vi "TDK多功能.vi"(0 "TDK地址":refnum<visa-resource-name>="COM15", 1 "工况1循环次数":i32, 2 "电源台数":dbl=3.0, 3 "工况1":string, 5 "工况切换地址":refnum<visa-resource-name>, 7 "工况2循环次数":i32, 9 "字符串":string, 10 "大循环次数":i32, 11 "错误输入（无错误）":errorcluster, 12 "工况地址":path, 13 "Bool引用句柄":refnum<vi>, 14 "工况2":string) -> (4 "运行总时间":dbl, 15 "错误输出":errorcluster)   [LabVIEW 2021]
uses:
  <vilib>/Utility/file.llb/Read Delimited Spreadsheet (DBL).vi
panel:
  out "?":string
  out "已成大循环数":i32
  in  "工况2":u16(ring) items=["新建 文本文档 (2)", "新建 文本文档 (3)", "新建 文本文档 (4)", "新建 文本文档"]
  in  "工况1":u16(ring) items=["新建 文本文档 (2)", "新建 文本文档 (3)", "新建 文本文档 (4)", "新建 文本文档"]
  out "?":u8(slide) scale=0.0..100.0
  out "电流":dbl(knob) scale=0.0..2000.0
  out "?":dbl[](graph)
  out "完成工况2循环":i32
  out "完成工况1循环":i32
  in  "延迟时间":dbl=1.0 caption="延迟时间(s)"
  in  "输入电流(A)":dbl
  in  "电流方向控制":cluster{"正向":bool, "反向":bool}
  out "?":bool
  out "?":bool
  in  "工况1":string[][](table)
  in  "工况2":string[][](table)
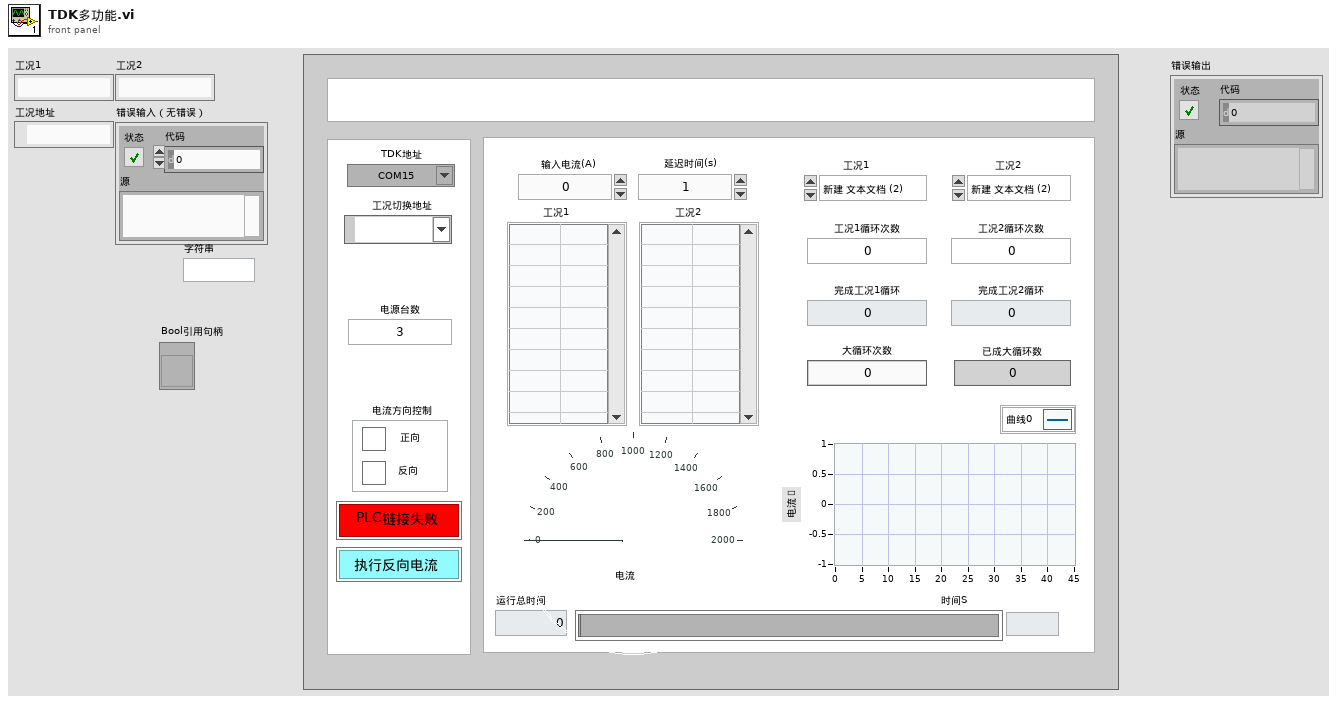
[diagram p1: front panel]
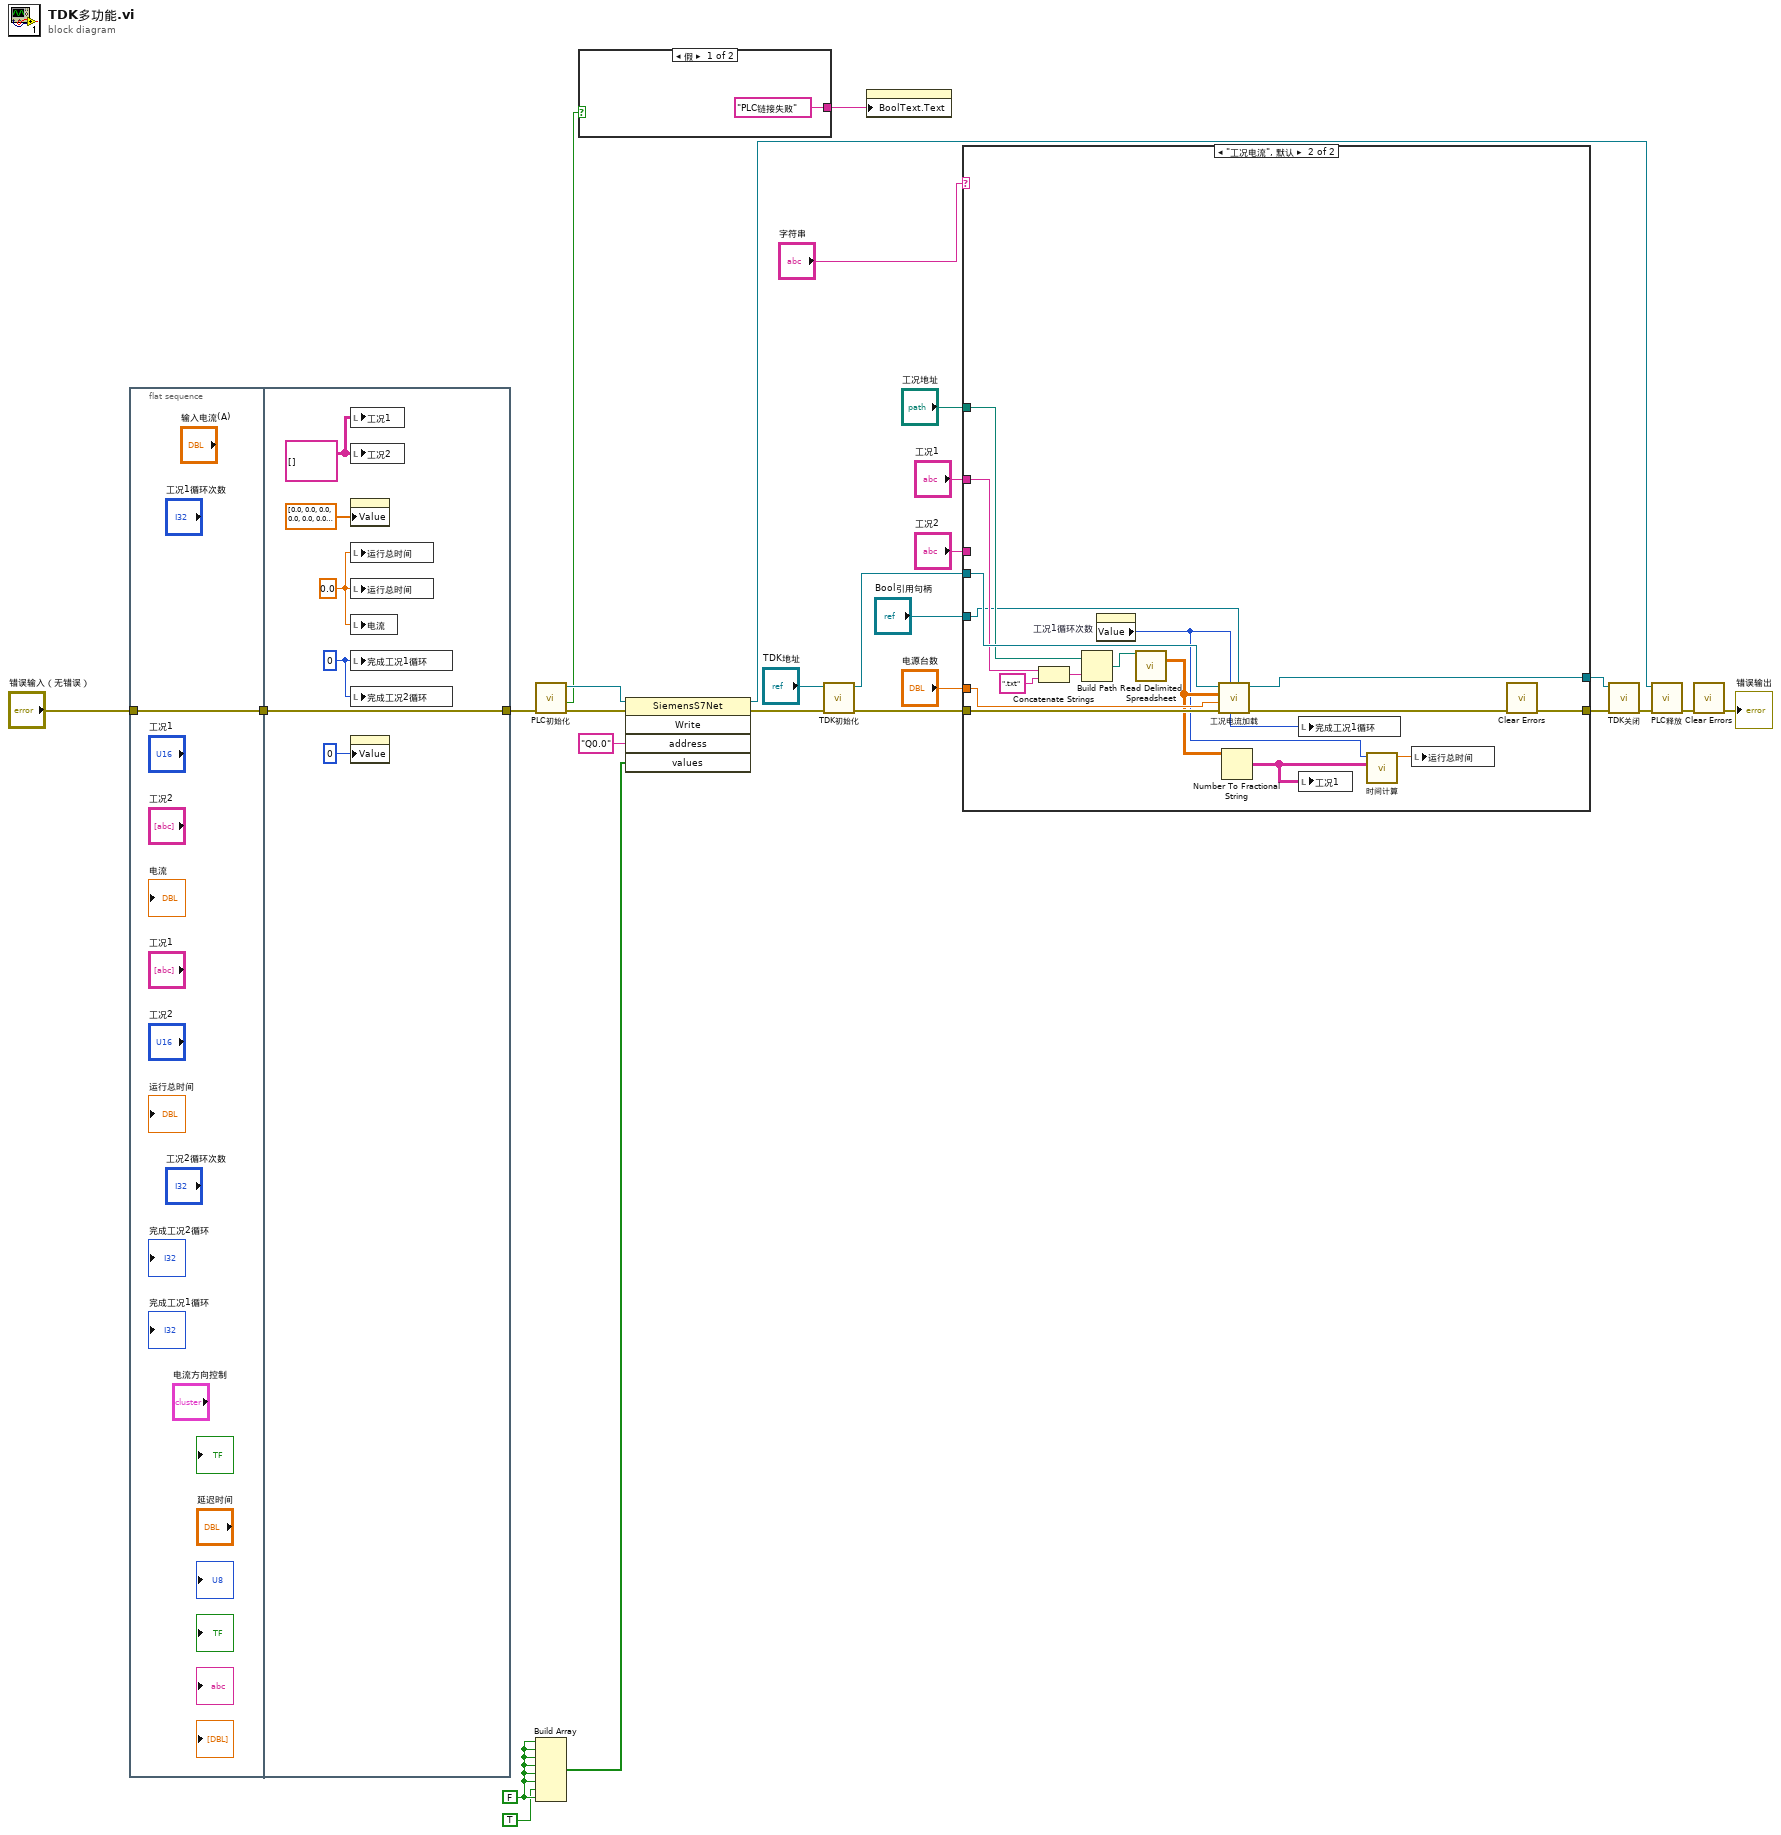
[diagram p0: block diagram]
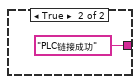
[diagram p2: hidden frame]
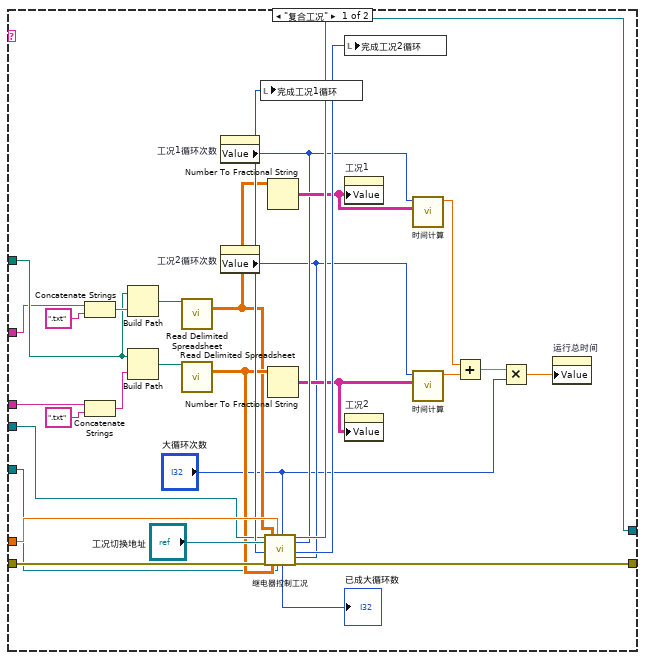
[diagram p3: hidden frame]
diagram:
  w11 = FALSE ("停止")
  n1 = flat-sequence {
    tunnel: "错误输入（无错误）" -> [w28]
    tunnel: [w28] -> w14
    tunnel: [w31] -> w8
    tunnel: w14 -> [w31]
    frame #0 {
    }
    frame #1 {
      w33 = 0
      w34 = string[][] [] ("工况1")
      w30 = 0.0
      n2 = local write "工况1"(w34) -> ()
      n3 = local write "工况2"(w34) -> ()
      n4 = property class="WFGraph (严格)"("Value"=dbl[] [0.0, 0.0, 0.0, 0.0, 0.0, 0.0, 0.0, 0.0, 0.0, 0.0, 0.0, 0.0, 0.0, 0.0, 0.0, 0.0, 0.0, 0.0, 0.0, 0.0, 0.0, 0.0, 0.0, 0.0, 0.0, 0.0, 0.0, 0.0, 0.0, 0.0, 0.0, 0.0, 0.0, 0.0, 0.0, 0.0, 0.0, 0.0, 0.0, 0.0, 0.0, 0.0, 0.0, 0.0, 0.0, 0.0]) -> ()  [unwired: 2 in, 2 out]
      n5 = local write "运行总时间"(w30) -> ()
      n6 = local write "运行总时间"(w30) -> ()
      n7 = local write "电流"(w30) -> ()
      n8 = local write "完成工况1循环"(w33) -> ()
      n9 = local write "完成工况2循环"(w33) -> ()
      n10 = property class="Slide (严格)"("Value"=u8 0) -> ()  [unwired: 2 in, 2 out]
    }
  }
  n11 = call "PLC初始化.vi"("错误输入（无错误）"=w8) -> ("错误输出"=w25:errorcluster, "IsSuccess"=w17:bool, "引用输出"=w26:refnum<k24>)  [unwired: 8 in]
  n12 = Build Array(w11, w11, w11, w11, w11, w11, TRUE ("元素"), w11) -> (w23:bool[])
  n13 = case shown="假" w17 {
    tunnel: ["PLC链接失败" "PLC链接成功"] -> w16
    frame False {
    }
    frame True {
    }
  }
  n14 = invoke class="SiemensS7Net" method="Write"(reference=w26, error in=w25, "address"="Q0.0", "values"=w23) -> (reference out=w20:refnum<k24>, error out=w24:errorcluster)  [unwired: 1 in, 3 out]
  n15 = call "TDK初始化.vi"("error in (no error)"=w24, "TDK地址"="TDK地址") -> ("error out"=w13:errorcluster, "VISA resource name out"=w15:refnum<visa-resource-name>)  [unwired: 8 in]
  n16 = property class="Bool (严格)"("BoolText.Text"=w16) -> ()  [unwired: 2 in, 2 out]
  n17 = case shown="\"工况电流\", 默认" "字符串" {
    tunnel: w15 -> [w58 w83]
    tunnel: [w62 w80] -> w18
    tunnel: w13 -> [w64 w81]
    tunnel: [w63 w74] -> w19
    tunnel: "电源台数" -> [w61 w82]
    tunnel: "工况地址" -> [w53 w77]
    tunnel: "工况1" -> [w39 w68]
    tunnel: "工况2" -> [w38 _]
    tunnel: "Bool引用句柄" -> [w37 w67]
    frame "复合工况" {
      n18 = Concatenate Strings(w39, ".txt" ("字符串")) -> (w54:string)
      n19 = Concatenate Strings(w38, ".txt" ("字符串")) -> (w57:string)
      n20 = Build Path(base path=w53, name or relative path=w54) -> (appended path=w50:path)
      n21 = Build Path(base path=w53, name or relative path=w57) -> (appended path=w52:path)
      n22 = call-poly <vilib>:"Read Delimited Spreadsheet.vi"("file path (dialog if empty)"=w50) -> ("all rows"=w49:dbl[][])  [unwired: 9 in, 5 out]
      n23 = call-poly <vilib>:"Read Delimited Spreadsheet.vi"("file path (dialog if empty)"=w52) -> ("all rows"=w51:dbl[][])  [unwired: 9 in, 5 out]
      n24 = property on="工况1循环次数" class="DigNum (严格)"() -> ("Value"=w47:i32)  [unwired: 2 in, 2 out]
      n25 = property on="工况2循环次数" class="DigNum (严格)"() -> ("Value"=w45:i32)  [unwired: 2 in, 2 out]
      n26 = call "继电器控制工况.vi"("tdk"=w58, "6332b"="工况切换地址", "error out"=w64, "工况1"=w49, "工况2"=w51, "电源台数"=w61, "Bool引用句柄"=w37, "大循环次数"="大循环次数", "工况1循环次数"=w47, "工况2循环次数"=w45) -> ("完成工况1循环"=w60:i32, "已成大循环数"=→"已成大循环数":i32, "VISA resource name out"=w62:refnum<visa-resource-name>, "完成工况2循环"=w59:i32, "错误输出"=w63:errorcluster)  [unwired: 5 in]
      n27 = local write "完成工况1循环"(w60) -> ()
      n28 = Number To Fractional String(number=w49) -> (F-format string=w48:string[][])  [unwired: 3 in]
      n29 = Number To Fractional String(number=w51) -> (F-format string=w46:string[][])  [unwired: 3 in]
      n30 = local write "完成工况2循环"(w59) -> ()
      n31 = property on="工况1" class="Tbl (严格)"("Value"=w48) -> ()  [unwired: 2 in, 2 out]
      n32 = property on="工况2" class="Tbl (严格)"("Value"=w46) -> ()  [unwired: 2 in, 2 out]
      n33 = call "时间计算.vi"("数组"=w48, "循环次数"=w47) -> ("x*y"=w44:dbl)  [unwired: 9 in]
      n34 = call "时间计算.vi"("数组"=w46, "循环次数"=w45) -> ("x*y"=w43:dbl)  [unwired: 9 in]
      n35 = Add(x=w44, y=w43) -> (x+y=w42:dbl)
      n36 = Multiply(x=w42, y="大循环次数") -> (x*y=w40:dbl)
      n37 = property on="运行总时间" class="DigNum (严格)"("Value"=w40) -> ()  [unwired: 2 in, 2 out]
    }
    frame "工况电流", Default {
      n38 = Concatenate Strings(w68, ".txt" ("字符串")) -> (w78:string)
      n39 = Build Path(base path=w77, name or relative path=w78) -> (appended path=w73:path)
      n40 = property on="工况1循环次数" class="DigNum (严格)"() -> ("Value"=w71:i32)  [unwired: 2 in, 2 out]
      n41 = call-poly <vilib>:"Read Delimited Spreadsheet.vi"("file path (dialog if empty)"=w73) -> ("all rows"=w72:dbl[][])  [unwired: 9 in, 5 out]
      n42 = call "工况电流加载.vi"("Bool引用句柄"=w67, "数值"=w71, "error in (no error)"=w81, "电源台数"=w82, "数组"=w72, "VISA resource name out"=w83) -> ("error out"=w75:errorcluster, "VISA resource name out 2"=w80:refnum<visa-resource-name>, "已完成循环"=w79:i32)  [unwired: 3 in]
      n43 = Number To Fractional String(number=w72) -> (F-format string=w70:string[][])  [unwired: 3 in]
      n44 = local write "完成工况1循环"(w79) -> ()
      n45 = local write "工况1"(w70) -> ()
      n46 = call "时间计算.vi"("数组"=w70, "循环次数"=w71) -> ("x*y"=w69:dbl)  [unwired: 9 in]
      n47 = local write "运行总时间"(w69) -> ()
      n48 = call <vilib>:"Clear Errors.vi"("error in (no error)"=w75) -> ("error out"=w74:errorcluster)  [unwired: 5 in, 1 out]
    }
  }
  n49 = call "TDK关闭.vi"("error in (no error)"=w19, "VISA resource name"=w18) -> ("error out"=w21:errorcluster)  [unwired: 9 in]
  n50 = call "PLC释放.vi"("错误输入（无错误） 2"=w21, "引用"=w20) -> ("错误输入（无错误）"=w12:errorcluster)  [unwired: 9 in]
  n51 = call <vilib>:"Clear Errors.vi"("error in (no error)"=w12) -> ("error out"=→"错误输出":errorcluster)  [unwired: 5 in, 1 out]
